vi "Аккумулятор4.vi"(1 "Reset":bool, 2 "C":bool, 3 "Enter":T2) -> (0 "Exit":T1)   [LabVIEW 2017]
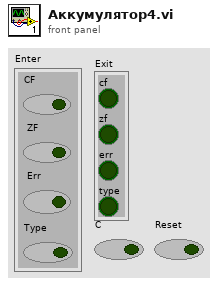
[diagram p1: front panel]
types:
  T1 = cluster{"cf":bool, "zf":bool, "err":bool, "type":bool}
  T2 = cluster{"CF":bool, "ZF":bool, "Err":bool, "Type":bool}
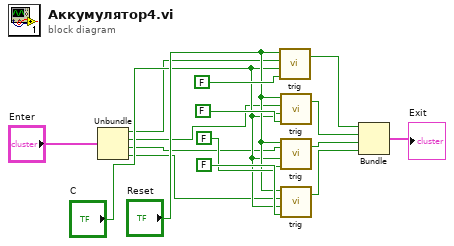
[diagram p0: block diagram]
diagram:
  n1 = Unbundle("Enter") -> ("CF"=w9:bool, "ZF"=w8:bool, "Err"=w7:bool, "Type"=w6:bool)
  n2 = call "trig.vi"("s"=FALSE, "c"="C", "d"=w9, "r"="Reset") -> ("q"=w2:bool)  [unwired: 1 out]
  n3 = call "trig.vi"("s"=FALSE, "c"="C", "d"=w8, "r"="Reset") -> ("q"=w3:bool)  [unwired: 1 out]
  n4 = call "trig.vi"("s"=FALSE, "c"="C", "d"=w7, "r"="Reset") -> ("q"=w4:bool)  [unwired: 1 out]
  n5 = call "trig.vi"("s"=FALSE, "c"="C", "d"=w6, "r"="Reset") -> ("q"=w5:bool)  [unwired: 1 out]
  n6 = Bundle("q"=w2, "q"=w3, "q"=w4, "q"=w5) -> (→"Exit":cluster{"q":bool, "q":bool, "q":bool, "q":bool})  [unwired: 1 in]
